vi "Invert_FFT_By_Harmonics.vi"(7 "signal In":waveform(dbl), 9 "phase f1-f9":dbl[](array[numeric])=[-2.296530890286755, -0.4996795442572583, 2.13231335701235, -2.8305146270300687, -3.0644603787657894, -1.910517808964867, -1.4604887262767599, -1.4608770943170013, -0.49288277337997893], 10 "mag f1-f9":dbl[](array[numeric])=[0.006255132621749245, 5.349180742819057e-10, 3.3971158138137566e-10, 2.020645150662673e-11, 3.443682420408273e-11, 3.747219651257019e-11, 4.2635827797213496e-11, 3.5893791114801e-11, 3.560739858812373e-11] format="%#_4p", 11 "Num Samp":dbl) -> (0 "dMdt":dbl[](graph), 2 "Summed Signal":waveform(dbl), 3 "Waveform Graph":waveform(dbl)[](graph))   [LabVIEW 2021]
uses:
  MPS_Labview/MPS_global_variables.vi
  <vilib>/measure/NI_MABase.lvlib
  <vilib>/Analysis/NI_AALPro.lvlib
panel:
  out "Waveform Graph 3":waveform(dbl)(graph)
  out "Waveform Graph 2":waveform(dbl)(graph)
  out "Drive Freq component":waveform(dbl)
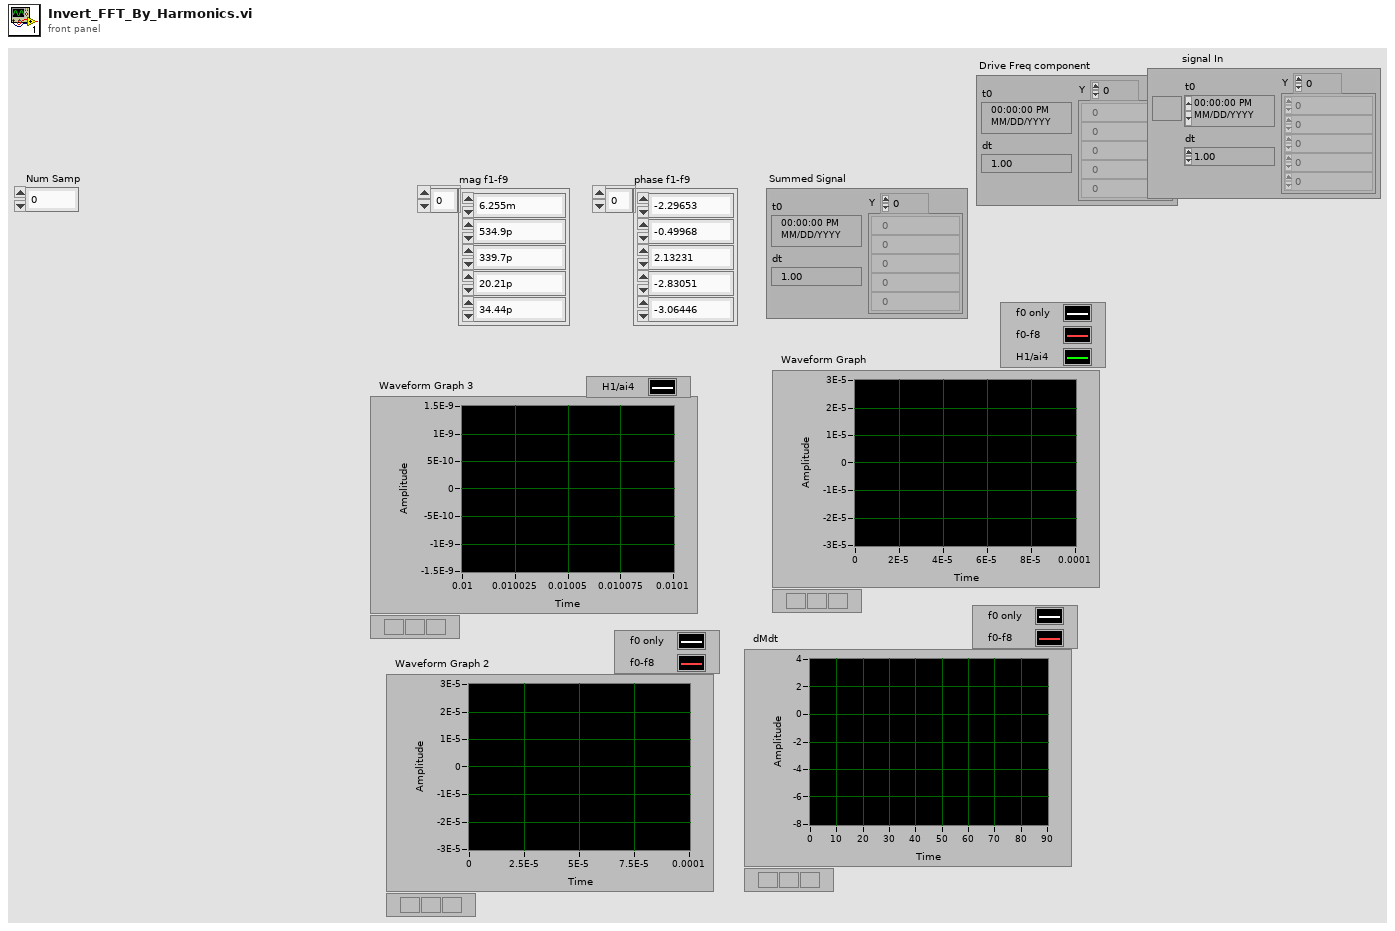
[diagram p1: front panel]
types:
  T1 = cluster{"sample rate":dbl, "Tx freq":dbl, "Tx amp":dbl, "Tx cycles\nSpectroscopy":dbl, "Bias amp":dbl, "Bias freq":dbl, "Receive range":dbl, "Bias Periods\nMagnetometry":dbl, "Tx Freq Division Factor":dbl, "Drive Periods per Bias":dbl, "TX harmonics":dbl[]}
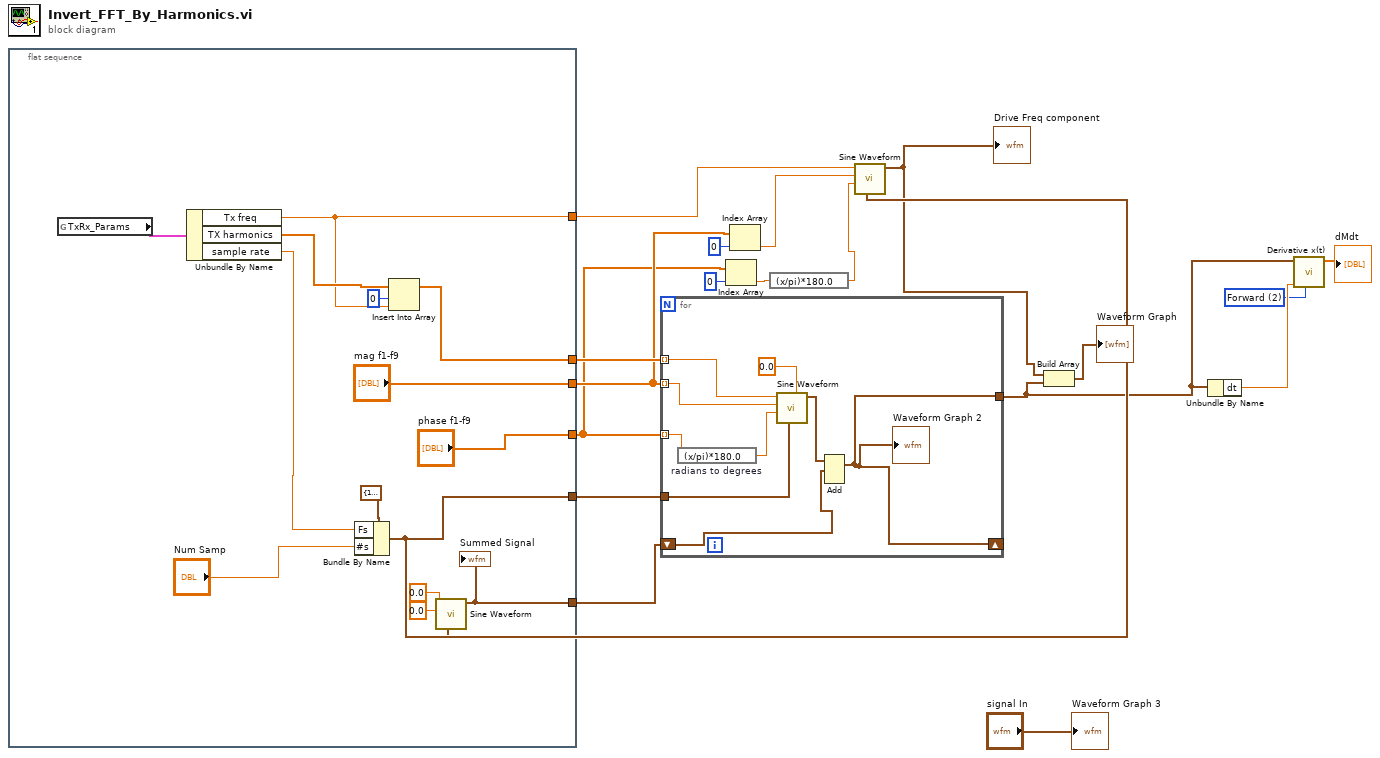
[diagram p0: block diagram]
diagram:
  w2 = u16 2 items=["2nd Order Central", "4th Order Central", "Forward", "Backward"] ("method")
  n1 = flat-sequence {
    tunnel: [w31] -> w18
    tunnel: [w23] -> w17
    tunnel: ["mag f1-f9"] -> w16
    tunnel: ["phase f1-f9"] -> w13
    tunnel: [w20] -> w11
    tunnel: [w19] -> w5
    frame #0 {
      n2 = global read "MPS_global_variables.vi" "TxRx_Params"() -> (w29:T1)
      n3 = Unbundle By Name(w29) -> ("Tx freq"=w23:dbl, "TX harmonics"=w28:dbl[], "sample rate"=w27:dbl)
      n4 = Bundle By Name(cluster=cluster{"Fs":dbl, "#s":dbl} {"Fs"=1000.0, "#s"=1000.0} ("sampling info"), "Fs"=w27, "#s"="Num Samp") -> (w20:cluster{"Fs":dbl, "#s":dbl})
      n5 = Insert Into Array(array=w28, index=0, new element=w23) -> (w31:dbl[])
      n6 = call <vilib>:"Sine Waveform.vi"("sampling info"=w20, "amplitude"=0.0, "frequency"=0.0) -> ("signal out"=w19:waveform(dbl))  [unwired: 7 in, 1 out]
      "Summed Signal" <- w19
    }
  }
  n7 = for {
    tunnel: w16 -> [w40] mode=indexing
    tunnel: w13 -> [w34] mode=indexing
    tunnel: w18 -> [w41] mode=indexing
    tunnel: w11 -> [w38]
    tunnel: [w35] -> w8
    shift-right: [w35] -> _
    shift-left: w5 -> [w36]
    n8 = expression code="(x/pi)*180.0" "radians to degrees"(w34) -> (w33:dbl)
    n9 = call <vilib>:"Sine Waveform.vi"("offset"=0.0, "sampling info"=w38, "phase"=w33, "amplitude"=w40, "frequency"=w41) -> ("signal out"=w37:waveform(dbl))  [unwired: 5 in, 1 out]
    n10 = Add(1:w36, 2:w37) -> (0:w35:waveform(dbl))  [unwired: 1 in, 1 out]
    "Waveform Graph 2" <- w35
  }
  n11 = Index Array(array=w13, index=0) -> (element=w4:dbl)
  n12 = Index Array(array=w16, index=0) -> (element=w12:dbl)
  n13 = expression code="(x/pi)*180.0" ("radians to degrees")(w4) -> (w3:dbl)
  n14 = call <vilib>:"Sine Waveform.vi"("sampling info"=w11, "phase"=w3, "amplitude"=w12, "frequency"=w17) -> ("signal out"=w10:waveform(dbl))  [unwired: 6 in, 1 out]
  "Drive Freq component" <- w10
  n15 = Build Array(w10, w8) -> (→"Waveform Graph":waveform(dbl)[])
  n16 = Unbundle By Name(w8) -> ("dt"=w7:dbl)
  n17 = call <vilib>:"Derivative x(t).vi"("method"=w2, "dt"=w7, "X"=w8) -> ("dX/dt"=→"dMdt":dbl[])  [unwired: 7 in, 1 out]
  "Waveform Graph 3" <- "signal In"
